vi "ScriptCommands.vi"(11 "Auton Routines":T1[](array[typedef])) -> ()   [LabVIEW 2014]
uses:
  Command Type.ctl
  <vilib>/Rock Robotics/WPI/DriverStation/DriverStationLCD/WPI_DriverStationLCDLCDLine.ctl
  Intake Actions.ctl
  <vilib>/Rock Robotics/WPI/RobotDrive/WPI_RobotDriveGetSetRefNum.vi
  Auto Pickup Global.vi
  Robot Global Data.vi
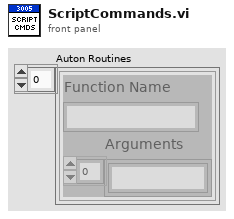
[diagram p1: front panel]
types:
  T1 = typedef "Command Type.ctl" = cluster{"Function Name":string, "Arguments":string[]}
  T2 = typedef "WPI_DriverStationLCDLCDLine.ctl" = enum16{"Main - Line 1", "User - Line 2", "User - Line 3", "User - Line 4", "User - Line 5", "User - Line 6"}
  T3 = typedef "Intake Actions.ctl" = enum16{"Extend", "Contain", "Motor Still", "Motor Outward", "Motor Inward", "Collect", "Pass", "Herd", "Contain Off", "Collect Delay Off", "Patea"}
  T4 = typedef "WPI_EncoderDevRef.ctl" = cluster{"DevStatus":errorcluster, "EncoderIndex":T5, "CounterIndex":T6, "DistancePerCount":dbl, "Decoding Type":T7}
  T5 = typedef "FPGA_EncoderIdx.ctl" = enum8{"Enc 0", "Enc 1", "Enc 2", "Enc 3", "Invalid"}
  T6 = typedef "FPGA_CounterCtrSystemIndex.ctl" = enum8{"Ctr 0", "Ctr 1", "Ctr 2", "Ctr 3", "Ctr 4", "Ctr 5", "Ctr 6", "Ctr 7", "Invalid"}
  T7 = typedef "WPI_EncoderType.ctl" = enum16{"1x", "2x", "4x"}
  T8 = typedef "WPI_RobotDriveDevRef.ctl" = cluster{"DevStatus":errorcluster, "Motors[]":T9[], "Square Inputs":bool, "Max Output":dbl}
  T9 = typedef "WPI_MotorControlDeviceRef.ctl" = cluster{"DeviceStatus":errorcluster, "Type":enum16{"PWM", "CAN"}, "PWM":cluster{"Digital Module":T10, "PWM Channel":T11, "DeadBand":T12}, "CAN":cluster{"Device Number":u8, "Control Mode":T13, "Semaphore":T14, "Max Vout":dbl}, "Invert":bool, "TransformRef":T15, "InvTransformRef":T15}
  T10 = typedef "FPGA_TypedefDigitalModule.ctl" = enum16{"Digital Module 1", "Digital Module 2"}
  T11 = typedef "FPGA_DIOPWMChannel.ctl" = enum8{"PWM 1", "PWM 2", "PWM 3", "PWM 4", "PWM 5", "PWM 6", "PWM 7", "PWM 8", "PWM 9", "PWM 10", "Invalid"}
  T12 = typedef "WPI_PWMDeadband.ctl" = cluster{"Name":string, "maxPositivePwm":i32, "minPositivePwm":i32, "centerPwm":i32, "maxNegativePwm":i32, "minNegativePwm":i32, "angularRange":u16}
  T13 = typedef "WPI_CANJaguar_ControlMode.ctl" = enum8{"Percent VBus", "Current", "Speed", "Position", "Voltage"}
  T14 = typedef "Semaphore RefNum" = refnum<k1>
  T15 = typedef "WPI_PWMTransform_ConPane.ctl" = refnum<vi>
  T16 = typedef "WPI_CounterDevRef.ctl" = cluster{"DevStatus":errorcluster, "CntIndex":T6}
  T17 = typedef "WPI_GyroDevRef.ctl" = cluster{"DevStatus":errorcluster, "Analog Module":T18, "Analog Channel":T19, "Offset":dbl, "Gain (VoltsPerDegree/Second)":dbl}
  T18 = typedef "FPGA_TypedefAnalogModule.ctl" = enum16{"Analog Module 1", "Analog Module 2"}
  T19 = typedef "FPGA_AIChannel.ctl" = enum8{"AI 1", "AI 2", "AI 3", "AI 4", "AI 5", "AI 6", "AI 7", "AI 8", "Invalid"}
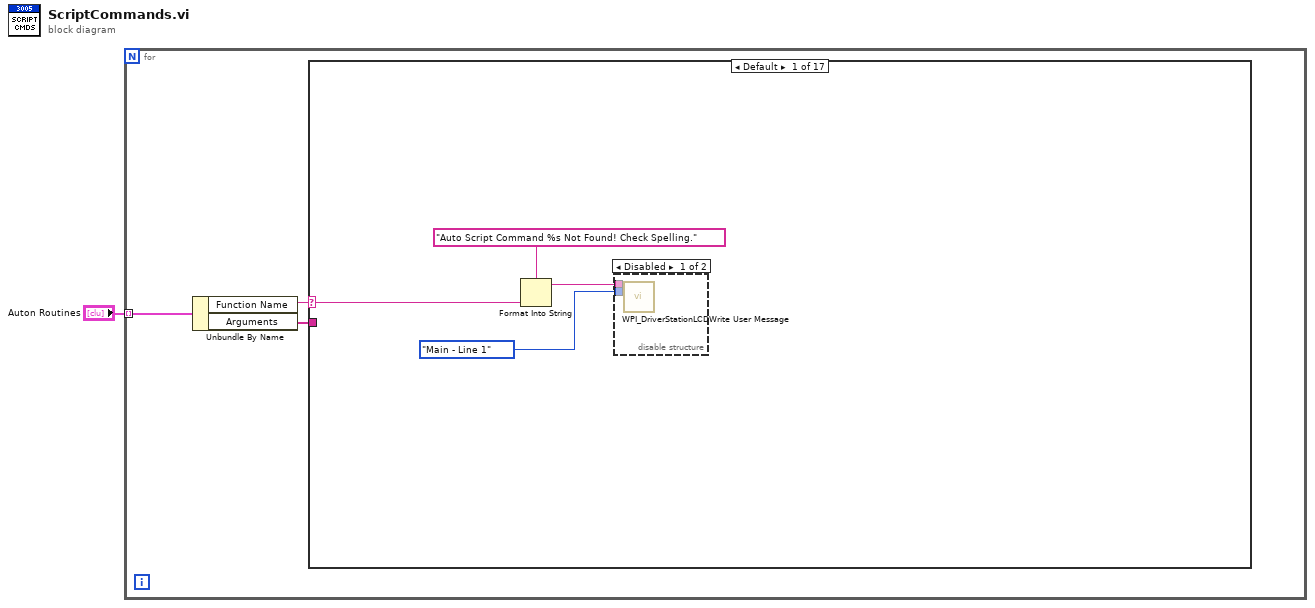
[diagram p0: block diagram]
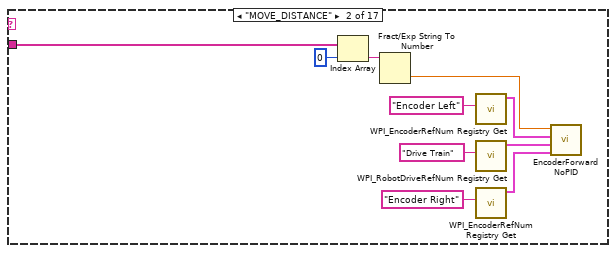
[diagram p3: hidden frame]
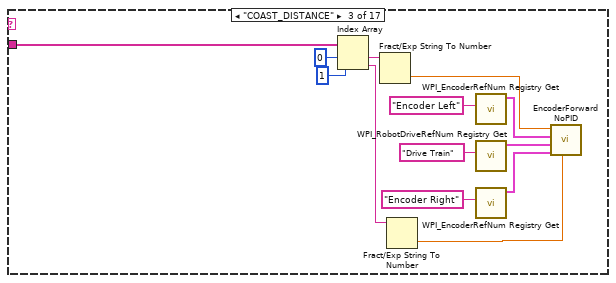
[diagram p4: hidden frame]
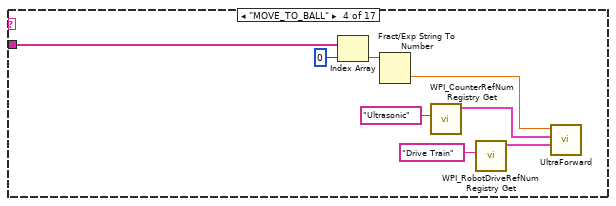
[diagram p5: hidden frame]
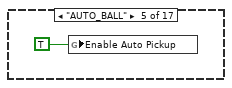
[diagram p6: hidden frame]
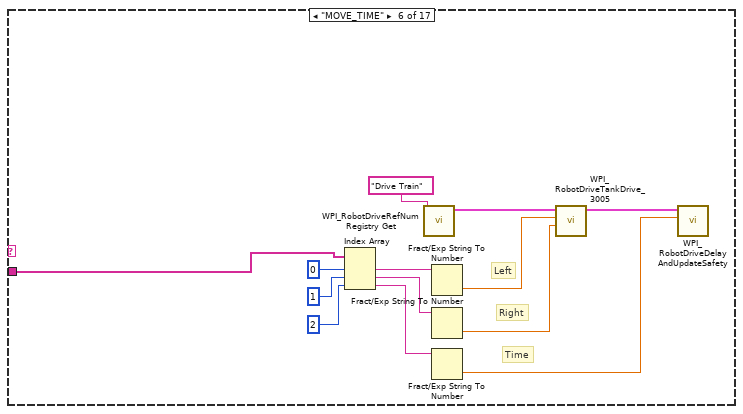
[diagram p7: hidden frame]
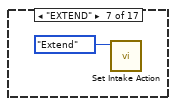
[diagram p8: hidden frame]
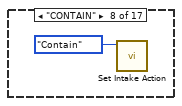
[diagram p9: hidden frame]
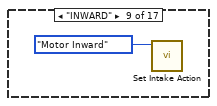
[diagram p10: hidden frame]
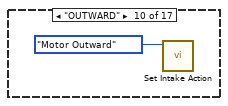
[diagram p11: hidden frame]
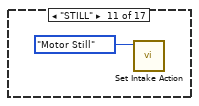
[diagram p12: hidden frame]
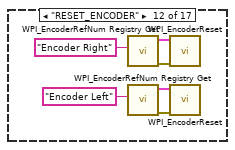
[diagram p13: hidden frame]
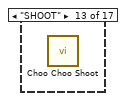
[diagram p14: hidden frame]
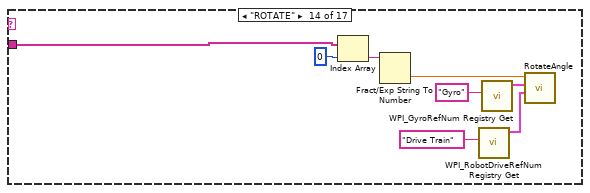
[diagram p15: hidden frame]
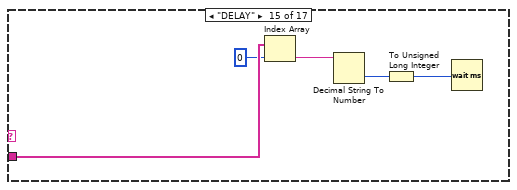
[diagram p16: hidden frame]
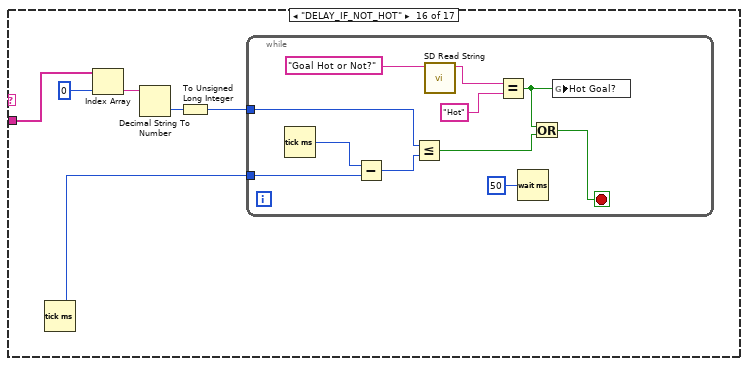
[diagram p17: hidden frame]
diagram:
  n1 = for {
    tunnel: "Auton Routines" -> [w4] mode=indexing
    n2 = Unbundle By Name(w4) -> ("Function Name"=w3:string, "Arguments"=w2:string[])
    n3 = case shown="Default" w3 {
      selector: w3 -> [w8 _ _ _ _ _ _ _ _ _ _ _ _ _ _ _ _]
      tunnel: w2 -> [_ w20 w33 w41 _ w43 _ _ _ _ _ _ _ w74 w79 w82 _]
      frame Default {
        n4 = Format Into String(format string="Auto Script Command %s Not Found! Check Spelling.", w8) -> (resulting string=w6:string)  [unwired: 2 in, 1 out]
        n5 = disable-structure shown="Disabled" {
          disable-tunnel: w6 -> [w10 _]
          disable-tunnel: WPI_DriverStationLCDLCDLine."Main - Line 1" ("line") -> [w9 _]
          frame Disabled {
            n6 = call <vilib>:"WPI_DriverStationLCDWrite User Message.vi"("line text"=w10, "line"=w9) -> ()  [unwired: 13 in, 1 out]
          }
          frame Enabled {
          }
        }
      }
      frame "MOVE_DISTANCE" {
        n7 = Index Array(array=w20, index=0) -> (element=w18:string)
        n8 = Fract/Exp String To Number(string=w18) -> (number=w11:dbl)  [unwired: 3 in, 1 out]
        n9 = call <vilib>:"WPI_EncoderRefNum Registry Get.vi"("refnum name"="Encoder Left") -> ("EncoderDevRef"=w12:T4)  [unwired: 9 in, 1 out]
        n10 = call <vilib>:"WPI_RobotDriveRefNum Registry Get.vi"("refnum name"="Drive Train") -> ("RobotDriveDevRef"=w16:T8)  [unwired: 1 in, 9 out]
        n11 = call <vilib>:"WPI_EncoderRefNum Registry Get.vi"("refnum name"="Encoder Right") -> ("EncoderDevRef"=w13:T4)  [unwired: 9 in, 1 out]
        n12 = call "EncoderForwardNoPID.vi"("EncoderDevRef 4"=w13, "RobotDriveDevRef"=w16, "EncoderDevRef"=w12, "Target"=w11) -> ()  [unwired: 5 in, 3 out]
      }
      frame "COAST_DISTANCE" {
        n13 = Index Array(array=w33, index #1=0 ("index"), index #2=1 ("index")) -> (element #1=w31:string, element #2=w22:string)
        n14 = Fract/Exp String To Number(string=w31) -> (number=w24:dbl)  [unwired: 3 in, 1 out]
        n15 = Fract/Exp String To Number(string=w22) -> (number=w23:dbl)  [unwired: 3 in, 1 out]
        n16 = call <vilib>:"WPI_EncoderRefNum Registry Get.vi"("refnum name"="Encoder Left") -> ("EncoderDevRef"=w25:T4)  [unwired: 9 in, 1 out]
        n17 = call <vilib>:"WPI_RobotDriveRefNum Registry Get.vi"("refnum name"="Drive Train") -> ("RobotDriveDevRef"=w29:T8)  [unwired: 1 in, 9 out]
        n18 = call <vilib>:"WPI_EncoderRefNum Registry Get.vi"("refnum name"="Encoder Right") -> ("EncoderDevRef"=w26:T4)  [unwired: 9 in, 1 out]
        n19 = call "EncoderForwardNoPID.vi"("Right axis value"=w23, "EncoderDevRef 4"=w26, "RobotDriveDevRef"=w29, "EncoderDevRef"=w25, "Target"=w24) -> ()  [unwired: 4 in, 3 out]
      }
      frame "MOVE_TO_BALL" {
        n20 = Index Array(array=w41, index=0) -> (element=w39:string)
        n21 = Fract/Exp String To Number(string=w39) -> (number=w36:dbl)  [unwired: 3 in, 1 out]
        n22 = call <vilib>:"WPI_CounterRefNum Registry Get.vi"("refnum name"="Ultrasonic") -> ("CounterDevRef"=w35:T16)  [unwired: 9 in, 1 out]
        n23 = call <vilib>:"WPI_RobotDriveRefNum Registry Get.vi"("refnum name"="Drive Train") -> ("RobotDriveDevRef"=w37:T8)  [unwired: 1 in, 9 out]
        n24 = call "UltraForward.vi"("RobotDriveDevRef"=w37, "CounterDevRef in"=w35, "Target"=w36) -> ()  [unwired: 8 in, 1 out]
      }
      frame "AUTO_BALL" {
        n25 = global write "Auto Pickup Global.vi" "Enable Auto Pickup"(TRUE ("Enable Auto Pickup")) -> ()
      }
      frame "MOVE_TIME" {
        # "Time"
        # "Right"
        # "Left"
        n26 = Index Array(array=w43, index #1=0 ("index"), index #2=1 ("index"), index #3=2 ("index")) -> (element #1=w49:string, element #2=w48:string, element #3=w47:string)
        n27 = call <vilib>:"WPI_RobotDriveRefNum Registry Get.vi"("refnum name"="Drive Train") -> ("RobotDriveDevRef"=w53:T8)  [unwired: 1 in, 9 out]
        n28 = Fract/Exp String To Number(string=w49) -> (number=w46:dbl)  [unwired: 3 in, 1 out]
        n29 = Fract/Exp String To Number(string=w48) -> (number=w45:dbl)  [unwired: 3 in, 1 out]
        n30 = Fract/Exp String To Number(string=w47) -> (number=w44:dbl)  [unwired: 3 in, 1 out]
        n31 = call <vilib>:"WPI_RobotDriveTankDrive_3005.vi"("Right axis value"=w45, "Left axis value"=w46, "RobotDriveDevRef"=w53) -> ("RobotDriveDevRef"=w55:T8)  [unwired: 6 in, 2 out]
        n32 = call <vilib>:"WPI_RobotDriveDelayAndUpdateSafety.vi"("Delay (s)"=w44, "RobotDriveDevRef"=w55) -> ()  [unwired: 8 in, 2 out]
      }
      frame "EXTEND" {
        n33 = call "Set Intake Action.vi"("Action"=Intake_Actions."Extend") -> ()  [unwired: 10 in, 1 out]
      }
      frame "CONTAIN" {
        n34 = call "Set Intake Action.vi"("Action"=Intake_Actions."Contain") -> ()  [unwired: 10 in, 1 out]
      }
      frame "INWARD" {
        n35 = call "Set Intake Action.vi"("Action"=Intake_Actions."Motor Inward") -> ()  [unwired: 10 in, 1 out]
      }
      frame "OUTWARD" {
        n36 = call "Set Intake Action.vi"("Action"=Intake_Actions."Motor Outward") -> ()  [unwired: 10 in, 1 out]
      }
      frame "STILL" {
        n37 = call "Set Intake Action.vi"("Action"=Intake_Actions."Motor Still") -> ()  [unwired: 10 in, 1 out]
      }
      frame "RESET_ENCODER" {
        n38 = call <vilib>:"WPI_EncoderRefNum Registry Get.vi"("refnum name"="Encoder Right") -> ("error out"=w66:errorcluster, "EncoderDevRef"=w65:T4)  [unwired: 9 in]
        n39 = call <vilib>:"WPI_EncoderRefNum Registry Get.vi"("refnum name"="Encoder Left") -> ("error out"=w61:errorcluster, "EncoderDevRef"=w62:T4)  [unwired: 9 in]
        n40 = call <vilib>:"WPI_EncoderReset.vi"("error in (no error)"=w66, "EncoderDevRef"=w65) -> ()  [unwired: 8 in, 2 out]
        n41 = call <vilib>:"WPI_EncoderReset.vi"("error in (no error)"=w61, "EncoderDevRef"=w62) -> ()  [unwired: 8 in, 2 out]
      }
      frame "SHOOT" {
        n42 = call "Choo Choo Shoot.vi"() -> ()  [unwired: 11 in, 1 out]
      }
      frame "ROTATE" {
        n43 = Index Array(array=w74, index=0) -> (element=w72:string)
        n44 = Fract/Exp String To Number(string=w72) -> (number=w67:dbl)  [unwired: 3 in, 1 out]
        n45 = call <vilib>:"WPI_RobotDriveRefNum Registry Get.vi"("refnum name"="Drive Train") -> ("RobotDriveDevRef"=w68:T8)  [unwired: 1 in, 9 out]
        n46 = call <vilib>:"WPI_GyroRefNum Registry Get.vi"("refnum name"="Gyro") -> ("GyroDevRef"=w71:T17)  [unwired: 9 in, 1 out]
        n47 = call "RotateAngle.vi"("RobotDriveDevRef"=w68, "GyroDevRef"=w71, "Target"=w67) -> ()  [unwired: 7 in, 2 out]
      }
      frame "DELAY" {
        n48 = Index Array(array=w79, index=0) -> (element=w77:string)
        n49 = Decimal String To Number(string=w77) -> (number=w76:i32)  [unwired: 2 in, 1 out]
        n50 = To Unsigned Long Integer(number=w76) -> (unsigned 32bit integer=w75:u32)
        n51 = Wait (ms)(milliseconds to wait=w75) -> ()  [unwired: 1 out]
      }
      frame "DELAY_IF_NOT_HOT" {
        n52 = Tick Count (ms)() -> (millisecond timer value=w81:u32)
        n53 = Index Array(array=w82, index=0) -> (element=w84:string)
        n54 = Decimal String To Number(string=w84) -> (number=w83:i32)  [unwired: 2 in, 1 out]
        n55 = To Unsigned Long Integer(number=w83) -> (unsigned 32bit integer=w80:u32)
        n56 = while {
          tunnel: w81 -> [w95]
          tunnel: w80 -> [w90]
          stop <- w87 stop-if-true
          n57 = Tick Count (ms)() -> (millisecond timer value=w94:u32)
          n58 = Subtract(x=w94, y=w95) -> (x-y=w93:u32)
          n59 = Less Or Equal?(x=w90, y=w93) -> (x <= y?=w92:bool)
          n60 = call <vilib>:"SD Read String.vi"("Name"="Goal Hot or Not?") -> ("String"=w89:string)  [unwired: 8 in, 2 out]
          n61 = Equal?(x=w89, y="Hot") -> (x = y?=w86:bool)
          n62 = Wait (ms)(milliseconds to wait=u32 50) -> ()  [unwired: 1 out]
          n63 = Or(x=w86, y=w92) -> (x .or. y?=w87:bool)
          n64 = global write "Robot Global Data.vi" "Hot Goal?"(w86) -> ()
        }
      }
      frame "STOP" {
      }
    }
  }
